vi "Dequeue.vi"(7 "Preview Queue (F)":bool, 8 "error in (no error)":errorcluster, 11 "MessageQueue":refnum<queue>) -> (0 "error out":errorcluster, 1 "Message Data":variant, 2 "Message":string, 3 "MessageQueue":refnum<queue>)   [LabVIEW 2018, in "SensorPlugins.lvlib"]
doc: "This VI removes and returns an element from the queue or returns an element from the queue without removing it from the queue."
uses:
  SensorPlugins.lvlib
  clMessage.ctl
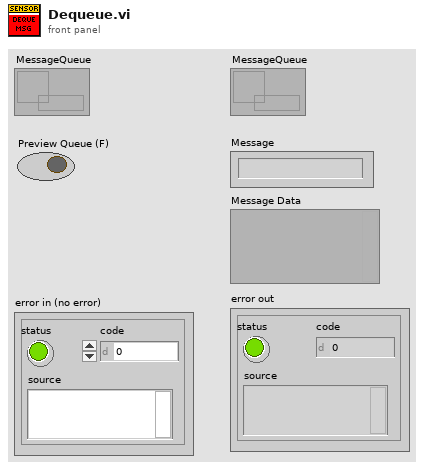
[diagram p1: front panel]
types:
  T1 = typedef "SensorPlugins.lvlib/clMessage.ctl" = cluster{"Message":string, "Message Data":variant}
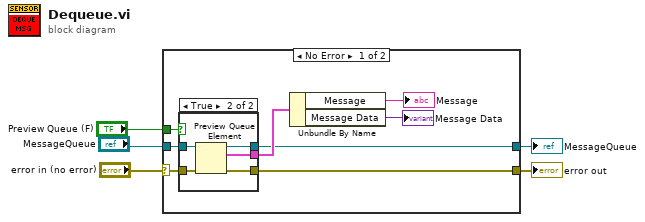
[diagram p0: block diagram]
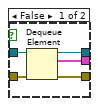
[diagram p2: hidden frame]
diagram:
  n1 = case shown="No Error" "error in (no error)" {
    selector: "error in (no error)" -> [w11 w24]
    tunnel: [w13 w24] -> w5
    tunnel: "MessageQueue" -> [w12 w25]
    tunnel: [w7 w25] -> w2
    tunnel: "Preview Queue (F)" -> [w6 _]
    frame No Error {
      n2 = case shown="True" w6 {
        tunnel: [w18 w23] -> w13
        tunnel: w12 -> [w17 w21]
        tunnel: w11 -> [w16 w22]
        tunnel: [w15 w19] -> w10
        tunnel: [w14 w20] -> w7
        frame False {
          n3 = Dequeue Element(queue=w17, error in (no error)=w16) -> (queue out=w14:refnum<queue>, element=w15:T1, error out=w18:errorcluster)  [unwired: 1 in, 1 out]
        }
        frame True {
          n4 = Preview Queue Element(queue=w21, error in (no error)=w22) -> (queue out=w20:refnum<queue>, element=w19:T1, error out=w23:errorcluster)  [unwired: 1 in, 1 out]
        }
      }
      n5 = Unbundle By Name(w10) -> ("Message"=→"Message":string, "Message Data"=→"Message Data":variant)
    }
    frame Error {
    }
  }
  "error out" <- w5
  "MessageQueue" <- w2
